vi "MainRe.vi"() -> ()   [LabVIEW 2019]
uses:
  <vilib>/robotics/Steering/Wheel/Wheel Parameters.ctl
  <vilib>/robotics/Steering/Wheel/Rotation Direction.ctl
  8e9cd874-ce80-48a6-9edb-c15c9fae371a.vi
  <vilib>/robotics/Steering/Fixed Wheel/NI_Robotics_Fixed Wheel.lvclass
  C:/Program Files (x86)/National Instruments/LabVIEW 2019/vi.lib/robotics/Steering/Wheel/NI_Robotics_Wheel.lvclass
  <vilib>/FPGAPlugInAG/myRIO-1900/niLvFpga_Open_myRIO-1900.vi
  <vilib>/rvi/interface/common/dynamic/niFpgaDynamicAddResources.vi
  <vilib>/Utility/error.llb/Error Cluster From Error Code.vi
  <vilib>/rvi/errors/niLvFpgaAdjustHostInterfaceError.vi
  <vilib>/robotics/Steering/Fixed Wheel/Create Fixed Wheel.vi
  <vilib>/robotics/Steering/Steering Frame/Create User Defined Steering Frame.vi
  <vilib>/FPGAPlugInAG/Dynamic/niLvFpga_Close_Dynamic.vi
  <vilib>/rvi/interface/nirviOpenFPGA/nirviOpenFPGA.xnode
  bitfiles/robotmecanum_FPGATarget_FPGAMainModified_RzoVAQMjhRw.lvbitx
  <vilib>/rvi/interface/nirviReadWriteControl/nirviReadWriteControl.xnode
  <vilib>/robotics/Steering/Create Steering Frame/NI_Robotics_Create Steering Frame.xnode
  <vilib>/robotics/Steering/Class Type Definitions/Steering Frame.ctl
  <vilib>/rvi/interface/nirviCloseFPGA/nirviCloseFPGA.xnode
  NiFpgaLv.dll
  <vilib>/rvi/interface/Simulation/niFpgaSimulationCallBeginRW.vi
  <vilib>/robotics/Steering/Steering Frame/NI_Robotics_Steering Frame.lvclass
  <vilib>/robotics/Steering/Class Type Definitions/NI_Robotics_Steering Class Types.lvlib
  <vilib>/robotics/Steering/Wheel/NI_Robotics_Wheel.lvclass
panel:
  in  "0, 1":i16
  in  "Test":dbl[](array[numeric])
  in  "Testing":bool
  out "EnVal":dbl[](array[numeric])
  in  "Numeric":u16
  out "Array 2":u16[](array[numeric])=[0, 1, 2, 3, 4, 5, 6, 7, 8, 9, 10, 11, 12, 13, 14, 15, 16, 17, 18, 19, 20, 21, 22, 23, 24, 25]
  in  "Array":T1(array[cluster])
  in  "Emergency":bool
  out "delay":i16
  out "VAL":dbl[](array[numeric])
  in  "Restart":bool
  in  "Start":bool
  in  "Run":i32
  in  "Stop":bool
  out "error out":errorcluster
  # "C/O"
  # "B/Y"
  # "A/X"
  # "Min"
  # "Mode"
  # "Max"
  # "Kp"
  # "B/Y"
  # "C/O"
  # "Mode"
  # "A/X"
  # "Sp"
  # "R-L"
  # "F-B"
  # "O"
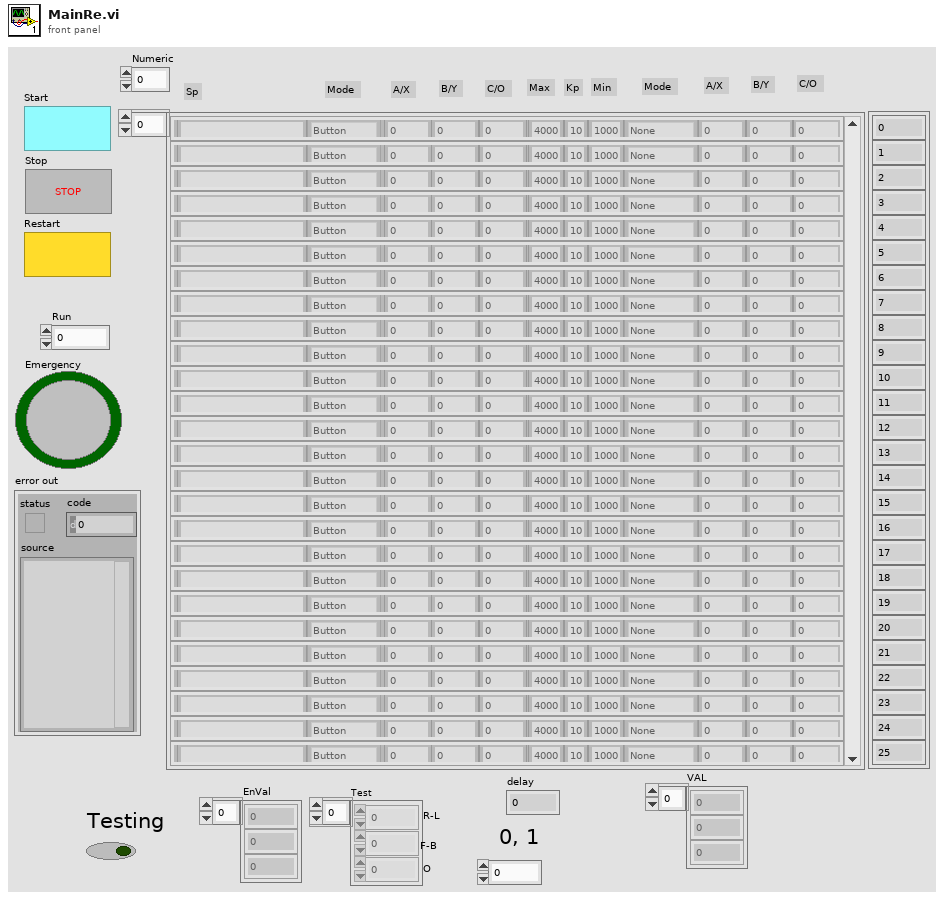
[diagram p1: front panel]
types:
  T1 = cluster{"Mode":enum16{"Button", "Encoder", "Delay", "IR Stop", "Line Stop"}, "A/X":dbl, "B/Y":dbl, "C/O":dbl, "Max":dbl, "Kp":dbl, "Min":dbl, "Mode 2":enum16{"None", "IR Stabilize", "Line Stabilize", "Encoder", "IR Stop", "Servo"}, "A/X 2":dbl, "B/Y 2":dbl, "C/O 2":dbl, "String":string}[]
  T2 = typedef "NI_Robotics_Wheel.lvclass/Wheel Parameters.ctl" = cluster{"wheel radius":dbl, "gear ratio":dbl, "forward rotation direction":T3}
  T3 = typedef "NI_Robotics_Wheel.lvclass/Rotation Direction.ctl" = u16
  T4 = typedef "NI_Robotics_Steering Class Types.lvlib/Steering Frame.ctl" = refnum<class "NI_Robotics_Steering Frame.lvclass">
  T5 = cluster{"Mode":enum16{"Button", "Encoder", "Delay", "IR Stop", "Line Stop"}, "A/X":dbl, "B/Y":dbl, "C/O":dbl, "Max":dbl, "Kp":dbl, "Min":dbl, "Mode 2":enum16{"None", "IR Stabilize", "Line Stabilize", "Encoder", "IR Stop", "Servo"}, "A/X 2":dbl, "B/Y 2":dbl, "C/O 2":dbl, "String":string}
  T6 = enum16{"None", "IR Stabilize", "Line Stabilize", "Encoder", "IR Stop", "Servo"}
  T7 = enum16{"Button", "Encoder", "Delay", "IR Stop", "Line Stop"}
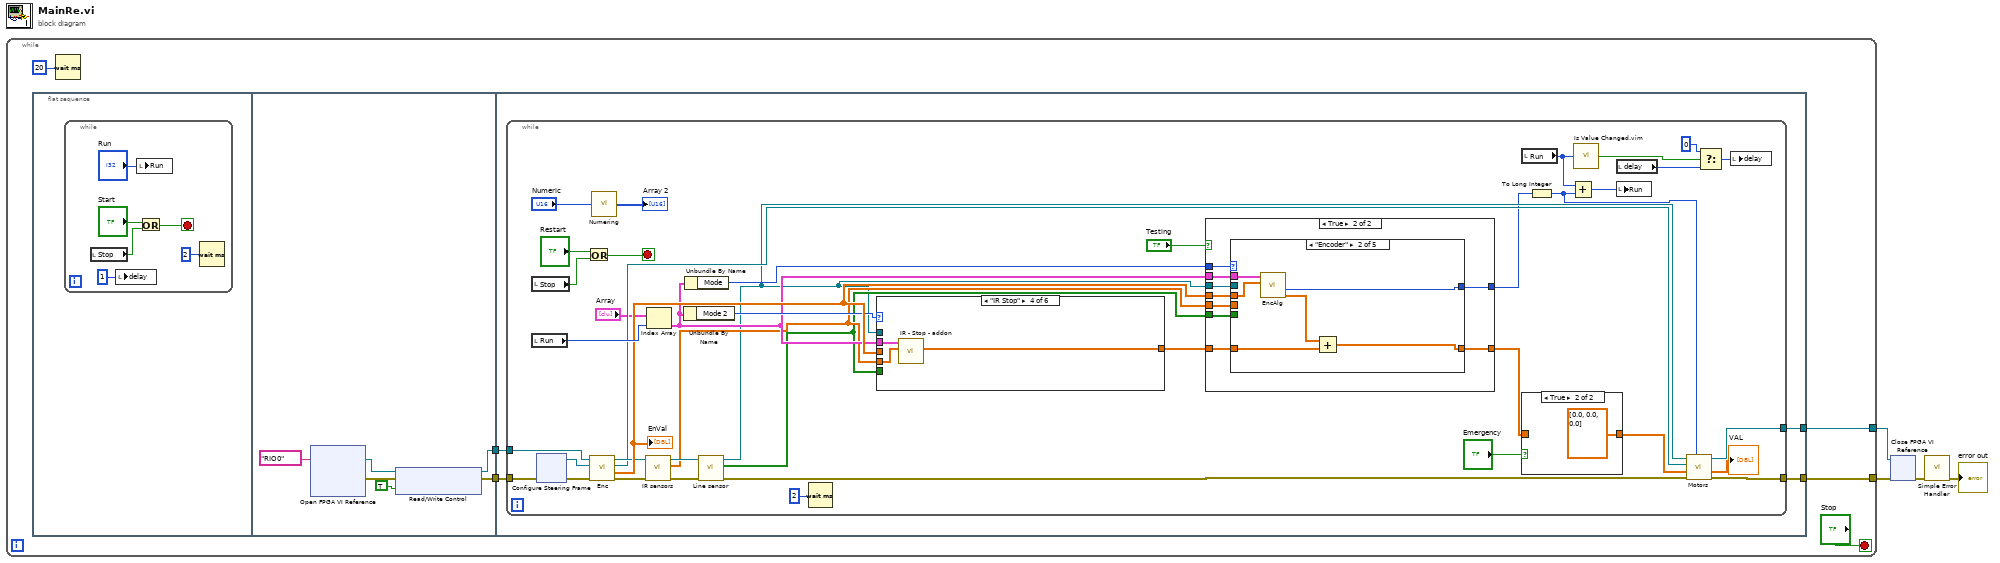
[diagram p0: block diagram]
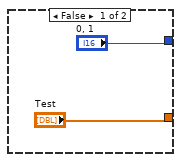
[diagram p2: hidden frame]
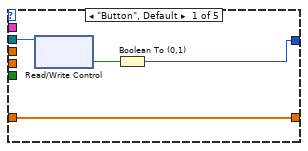
[diagram p3: hidden frame]
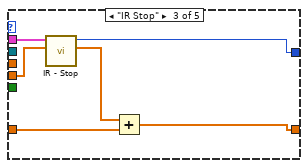
[diagram p4: hidden frame]
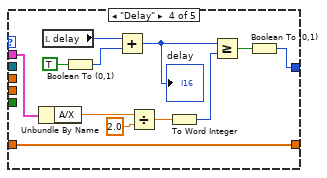
[diagram p5: hidden frame]
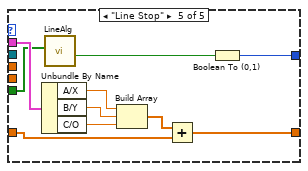
[diagram p6: hidden frame]
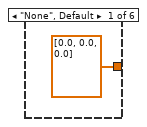
[diagram p7: hidden frame]
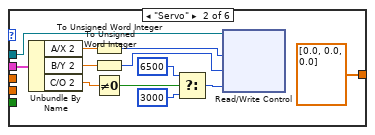
[diagram p8: hidden frame]
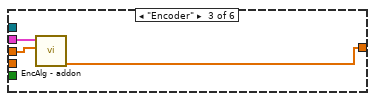
[diagram p9: hidden frame]
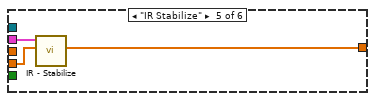
[diagram p10: hidden frame]
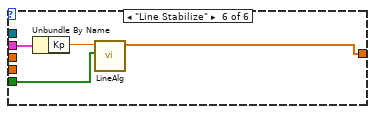
[diagram p11: hidden frame]
diagram:
  n1 = while {
    tunnel: [w8] -> w2
    tunnel: [w7] -> w1
    stop <- "Stop" stop-if-true
    n2 = flat-sequence {
      tunnel: [w19] -> w10
      tunnel: [w18] -> w9
      tunnel: w10 -> [w26]
      tunnel: w9 -> [w23]
      tunnel: [w25] -> w8
      tunnel: [w24] -> w7
      frame #0 {
        n3 = while {
          stop <- w12 stop-if-true
          n4 = local read "Stop"() -> (w11:bool)
          n5 = local write "delay"(i16 1 ("delay")) -> ()
          n6 = local write "Run"("Run") -> ()
          n7 = Or(x="Start", y=w11) -> (x .or. y?=w12:bool)
          n8 = Wait (ms)(milliseconds to wait=u32 2) -> ()  [unwired: 1 out]
        }
      }
      frame #1 {
        n9 = xnode "Open FPGA VI Reference"("resource name"=tag "RIO0") -> ("FPGA VI Reference Out"=w22:refnum<k20>, "error out"=w20:errorcluster)  [unwired: 1 in]
        n10 = xnode "Read/Write Control"("FPGA VI Reference In"=w22, "error in"=w20, "RESET ENCODER"=TRUE) -> ("FPGA VI Reference Out"=w19:refnum<k20>, "error out"=w18:errorcluster)
      }
      frame #2 {
        n11 = while {
          tunnel: w26 -> [w66]
          tunnel: [w61] -> w25
          tunnel: [w60] -> w24
          tunnel: w23 -> [w30]
          stop <- w37 stop-if-true
          n12 = local read "Stop"() -> (w35:bool)
          n13 = local read "Run"() -> (w65:i32)
          n14 = xnode ("Configure Steering Frame")("error in (no error)"=w30) -> ("steering frame out"=w29:T4, "error out"=w31:errorcluster)
          n15 = Or(x="Restart", y=w35) -> (x .or. y?=w37:bool)
          n16 = call "Enc.vi"("FPGA VI Reference In"=w66, "steering frame in"=w29, "error in"=w31) -> ("FPGA VI Reference Out"=w59:refnum<k20>, "steering frame out"=w50:T4, "EnVal"=w63:dbl[], "error out"=w58:errorcluster)  [unwired: 4 in]
          "EnVal" <- w63
          n17 = call "Numering.vi"("Numeric"="Numeric") -> ("Array 2"=→"Array 2":u16[])
          n18 = call "IR sensors.vi"("error in"=w58, "FPGA VI Reference In"=w59) -> ("error out"=w57:errorcluster, "IR Sensors"=w52:dbl[], "FPGA VI Reference Out"=w56:refnum<k20>)  [unwired: 7 in]
          n19 = Index Array(array="Array", index=w65) -> (element=w53:T5)
          n20 = Unbundle By Name(w53) -> ("Mode 2"=w54:T6)
          n21 = Unbundle By Name(w53) -> ("Mode"=w64:T7)
          n22 = call "Line sensor.vi"("error in"=w57, "FPGA VI Reference In"=w56) -> ("error out"=w55:errorcluster, "appended array"=w51:bool[], "FPGA VI Reference Out"=w48:refnum<k20>)  [unwired: 7 in]
          n23 = Wait (ms)(milliseconds to wait=u32 2) -> ()  [unwired: 1 out]
          n24 = case shown="\"IR Stop\"" w54 {
            tunnel: [dbl[] [0.0, 0.0, 0.0] ("y") dbl[] [0.0, 0.0, 0.0] ("appended array") w131 w133 w136 w139] -> w28
            tunnel: w53 -> [_ w127 w132 w135 w138 w142]
            tunnel: w52 -> [_ _ _ w134 w137 _]
            tunnel: w51 -> [_ _ _ _ _ w140]
            tunnel: w63 -> [_ _ w130 _ _ _]
            tunnel: w48 -> [_ w129 _ _ _ _]
            frame "None", Default {
            }
            frame "Servo" {
              n25 = Unbundle By Name(w127) -> ("A/X 2"=w126:dbl, "B/Y 2"=w123:dbl, "C/O 2"=w122:dbl)
              n26 = To Unsigned Word Integer(number=w126) -> (unsigned 16bit integer=w125:u16)
              n27 = To Unsigned Word Integer(number=w123) -> (unsigned 16bit integer=w124:u16)
              n28 = Not Equal To 0?(x=w122) -> (x != 0?=w121:bool)
              n29 = Select(t=u16 6500 ("SERVO 3"), s=w121, f=u16 3000 ("SERVO 3")) -> (s? t:f=w120:u16)
              n30 = xnode "Read/Write Control"("FPGA VI Reference In"=w129, "SERVO 1"=w125, "SERVO 2"=w124, "SERVO 3"=w120) -> ()  [unwired: 1 in, 2 out]
            }
            frame "Encoder" {
              n31 = call "EncAlg - addon.vi"("EnValIn"=w130, "element"=w132) -> ("VelValOut"=w131:dbl[])  [unwired: 7 in, 2 out]
            }
            frame "IR Stop" {
              n32 = call "IR - Stop - addon.vi"("IR Sensors"=w134, "element"=w135) -> ("appended array"=w133:dbl[])  [unwired: 8 in, 1 out]
            }
            frame "IR Stabilize" {
              n33 = call "IR - Stabilize.vi"("IR Sensors"=w137, "element"=w138) -> ("appended array"=w136:dbl[])  [unwired: 8 in, 1 out]
            }
            frame "Line Stabilize" {
              n34 = Unbundle By Name(w142) -> ("Kp"=w141:dbl)
              n35 = call "LineAlg.vi"("array"=w140, "Kp"=w141) -> ("appended array"=w139:dbl[])  [unwired: 8 in, 1 out]
            }
          }
          n36 = case shown="True" "Testing" {
            tunnel: w64 -> [_ w78]
            tunnel: w63 -> [_ w77]
            tunnel: w53 -> [_ w76]
            tunnel: w52 -> [_ w75]
            tunnel: w51 -> [_ w74]
            tunnel: w48 -> [_ w73]
            tunnel: ["0, 1" w72] -> w46
            tunnel: ["Test" w71] -> w38
            tunnel: w28 -> [_ w70]
            frame False {
            }
            frame True {
              n37 = case shown="\"Encoder\"" w78 {
                tunnel: w76 -> [_ w88 w94 w106 w116]
                tunnel: w77 -> [_ w87 _ _ _]
                tunnel: [w79 w86 w91 w95 w113] -> w71
                tunnel: w70 -> [w79 w85 w93 w95 w112]
                tunnel: [w80 w84 w90 w105 w108] -> w72
                tunnel: w73 -> [w82 _ _ _ _]
                tunnel: w75 -> [_ _ w89 _ _]
                tunnel: w74 -> [_ _ _ _ w114]
                frame "Button", Default {
                  n38 = xnode "Read/Write Control"("FPGA VI Reference In"=w82) -> ("C DIO 0"=w81:bool)  [unwired: 1 in, 2 out]
                  n39 = Boolean To (0,1)(Boolean=w81) -> (0, 1=w80:i16)
                }
                frame "Encoder" {
                  n40 = call "EncAlg.vi"("EnValIn"=w87, "element"=w88) -> ("VelValOut"=w83:dbl[], "0, 1"=w84:i16)  [unwired: 7 in, 1 out]
                  n41 = Add(x=w83, y=w85) -> (x+y=w86:dbl[])
                }
                frame "IR Stop" {
                  n42 = call "IR - Stop.vi"("IR Sensors"=w89, "element"=w94) -> ("appended array"=w92:dbl[], "0, 1"=w90:i16)  [unwired: 8 in]
                  n43 = Add(x=w92, y=w93) -> (x+y=w91:dbl[])
                }
                frame "Delay" {
                  n44 = Unbundle By Name(w106) -> ("A/X"=w101:dbl)
                  n45 = local read "delay"() -> (w102:i16)
                  n46 = Boolean To (0,1)(Boolean=TRUE) -> (0, 1=w103:i16)
                  n47 = Add(x=w102, y=w103) -> (x+y=w97:i16)
                  "delay" <- w97
                  n48 = Divide(x=w101, y=2.0) -> (x/y=w99:dbl)
                  n49 = To Word Integer(number=w99) -> (16bit integer=w98:i16)
                  n50 = Greater Or Equal?(x=w97, y=w98) -> (x >= y?=w96:bool)
                  n51 = Boolean To (0,1)(Boolean=w96) -> (0, 1=w105:i16)
                }
                frame "Line Stop" {
                  n52 = Unbundle By Name(w116) -> ("A/X"=w111:dbl, "B/Y"=w110:dbl, "C/O"=w109:dbl)
                  n53 = call "LineAlg.vi"("array"=w114) -> ("logical OR"=w115:bool)  [unwired: 9 in, 1 out]
                  n54 = Build Array(w111, w110, w109) -> (w107:dbl[])
                  n55 = Add(x=w107, y=w112) -> (x+y=w113:dbl[])
                  n56 = Boolean To (0,1)(Boolean=w115) -> (0, 1=w108:i16)
                }
              }
            }
          }
          n57 = local read "Run"() -> (w45:i32)
          n58 = case shown="True" "Emergency" {
            tunnel: [w162 dbl[] [0.0, 0.0, 0.0] ("VelValIn")] -> w39
            tunnel: w38 -> [w162 _]
            frame False {
            }
            frame True {
            }
          }
          n59 = To Long Integer(number=w46) -> (32bit integer=w49:i32)
          n60 = Add(x=w45, y=w49) -> (x+y=w62:i32)
          n61 = call "Is Value Changed.vim"("value"=w45) -> ("changed or first call?"=w44:bool)
          n62 = local read "delay"() -> (w43:i16)
          n63 = local write "Run"(w62) -> ()
          n64 = call "Motors.vi"("x"=w49, "error in (no error)"=w55, "VelValIn"=w39, "steering frame in"=w50, "FPGA VI Reference In"=w48) -> ("error out"=w60:errorcluster, "VAL"=→"VAL":dbl[], "FPGA VI Reference  out"=w61:refnum<k20>)  [unwired: 3 in, 1 out]
          n65 = Select(t=i16 0, s=w44, f=w43) -> (s? t:f=w41:i16)
          n66 = local write "delay"(w41) -> ()
        }
      }
    }
    n67 = Wait (ms)(milliseconds to wait=u32 20) -> ()  [unwired: 1 out]
  }
  n68 = xnode "Close FPGA VI Reference"("FPGA VI Reference In"=w2, "error in"=w1) -> ("error out"=w3:errorcluster)
  n69 = call <vilib>:"Simple Error Handler.vi"("error in (no error)"=w3) -> ("error out"=→"error out":errorcluster)  [unwired: 4 in, 4 out]
